vi "sub_log-img.vi"(8 "error in (no error)":errorcluster caption="error in") -> (0 "error out":errorcluster)   [LabVIEW 2019]
uses:
  logfile-name.vi
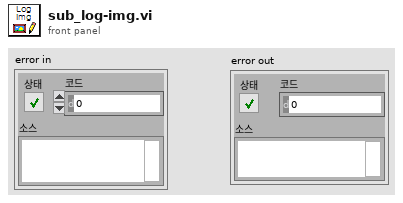
[diagram p1: front panel]
types:
  T1 = typedef "IMAQ Image.ctl" = refnum<image>
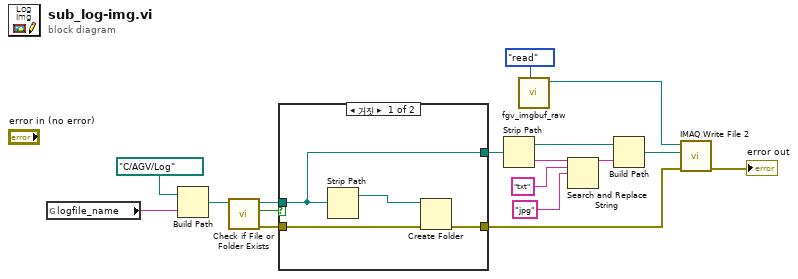
[diagram p0: block diagram]
diagram:
  n1 = global read "logfile-name.vi" "logfile_name"() -> (w12:string)
  n2 = Build Path(base path=path "C:/AGV/Log" ("베이스 경로"), name or relative path=w12) -> (appended path=w14:path)
  n3 = call <vilib>:"Check if File or Folder Exists.vi"("path"=w14) -> ("error out"=w13:errorcluster, "file or folder exists?"=w15:bool, "dup path"=w16:path)  [unwired: 8 in]
  n4 = case shown="거짓" w15 {
    tunnel: w16 -> [w20 w23]
    tunnel: [w20 w23] -> w7
    tunnel: w13 -> [w19 w22]
    tunnel: [w18 w22] -> w8
    frame False {
      n5 = Strip Path(path=w20) -> (stripped path=w21:path)  [unwired: 1 out]
      n6 = Create Folder(path (use dialog)=w21, error in=w19) -> (error out=w18:errorcluster)  [unwired: 1 in, 2 out]
    }
    frame True {
    }
  }
  n7 = Strip Path(path=w7) -> (stripped path=w6:path, name=w4:string)
  n8 = call "fgv_imgbuf_raw.vi"("cmd"=enum16{"create", "close", "write", "read"}."read") -> ("Image"=w10:T1)  [unwired: 9 in, 1 out]
  n9 = Search and Replace String(input string=w4, search string="txt" ("검색 문자열"), replace string="jpg" ("이름 또는 상대 경로")) -> (result string=w1:string)  [unwired: 5 in, 3 out]
  n10 = Build Path(base path=w6, name or relative path=w1) -> (appended path=w5:path)
  n11 = call-poly "IMAQ Write File 2"("error in (no error)"=w8, "File Path"=w5, "Image"=w10) -> ("error out"=→"error out":errorcluster)  [unwired: 7 in, 1 out]
